vi "Pointer producer consumer Read Write Serial Port.vi"(7 "write string":string, 8 "error in (no error)":errorcluster, 11 "VISA resource name out":refnum<visa-resource-name>) -> (0 "error out":errorcluster, 1 "timeout?":bool, 2 "read string":string, 3 "bytes read":u32)   [LabVIEW 2014]
doc: "The Basic Serial Read and Write example performs a Serial Port Read, a Serial Port Write, or a combination of these actions. The user selects the actions (read or write) on the front panel. If both are selected, the VI will write the data first, read data, and then close the VISA session that is opened to the port. This VI will wait until the specified number of bytes is received at the port or until a termination character is read.\n\nINSTRUCTIONS:\n1) Select the serial resource and configuration parameters (baud rate, data bits, parity, stop bits, flow control).\n2) Select the operations to be performed. \n3) Connect the serial port to your device. If no device is available, perform a loopback test by doing one of the following. Short pins 2 and 3 on a RS-232 cable or short pin 4 to pin 8 and pin 5 to pin 9 on a RS-485/422 cable. \n4) Run the VI to see the data read. (The \"read string\" will match the \"string to write\" if a loopback test was performed.)\n\nNote: The parameters set for the serial port must match the parameters of the connected instrument or device. In this example, the bytes to read parameter specifies the number of bytes that the serial port reads. If there were more bytes at the port than the number specified in bytes to read, those bytes would not be read. Also, if you specify to read more bytes than the number of bytes actually read, you might receive a timeout error message.\n\nOn the block diagram, the Configure Serial Port VI sets the configuration parameters. The front panel displays the controls used to configure the basic parameters, such as baud rate, data bits, and parity. Constants configure the other parameters the user probably does not need set. After the VISA Configure Serial Port VI opens the VISA session and configures the port, the VI passes the VISA resource name to other VIs that perform operations on that VISA resource. The VISA Write function sends a command to the serial device and the VISA Read function returns data based on the command. The VISA Close function then closes the reference to the serial device. It is important to close the reference; otherwise communication through with that port through protocols other than VISA might not be possible."
uses:
  <vilib>/Instr/_visa.llb/VISA Flush IO Buffer Mask.ctl
panel:
  out "comm time":u32
  # "Select the serial resource and the operations (Read, Write, or both) to be performed.  If both are selected, the VI will write the data first, read data and then close the VISA session that is opened to the port.  This VI will wait until the specified number of bytes is received at the port or until a termination character is read."
  # "For additional information select File >> VI Properties >> Documentation"
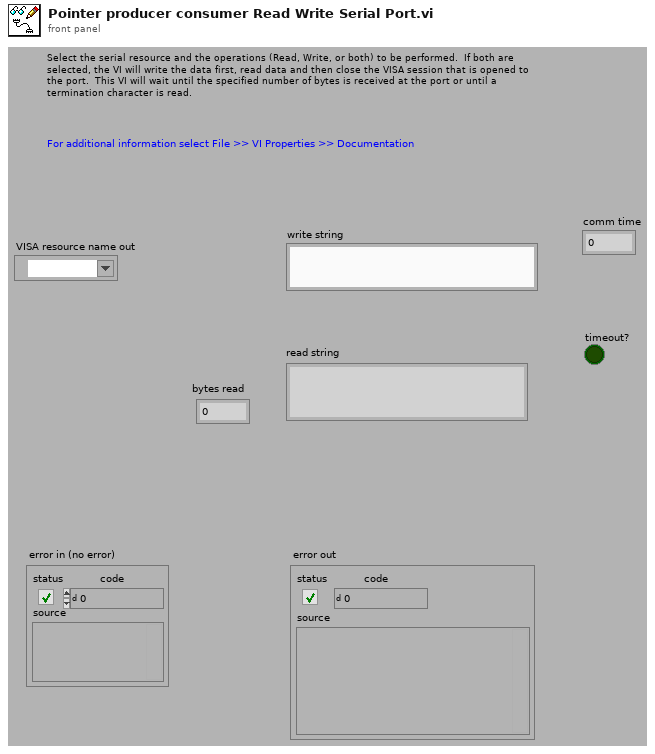
[diagram p1: front panel]
types:
  T1 = typedef "VISA Flush IO Buffer Mask.ctl" = u16
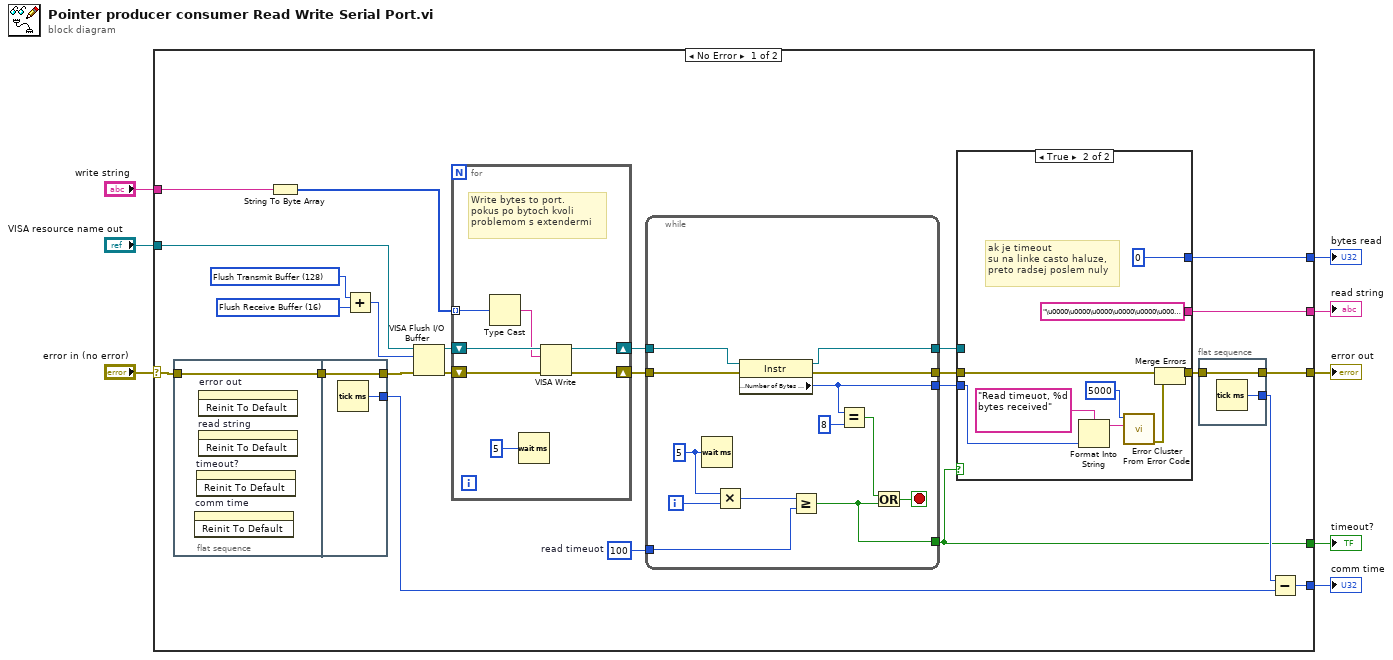
[diagram p0: block diagram]
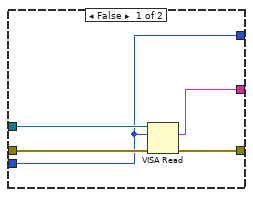
[diagram p2: hidden frame]
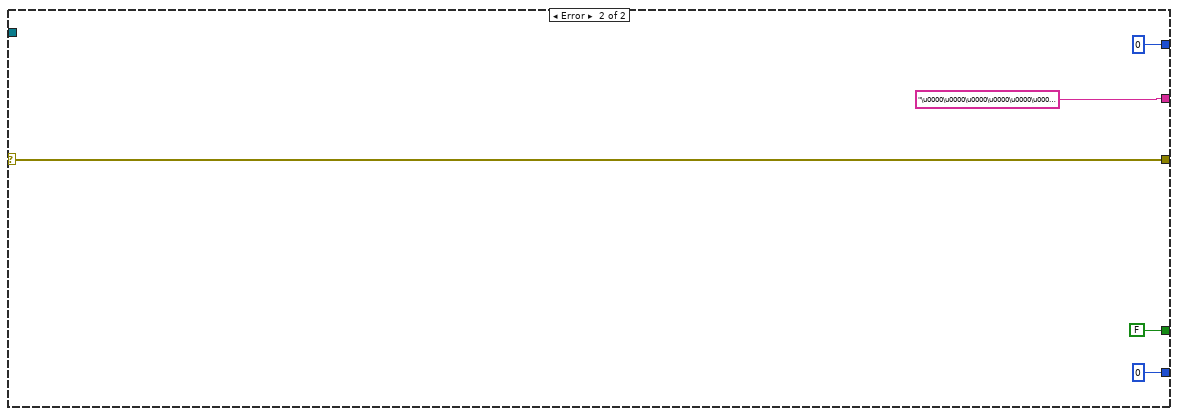
[diagram p3: hidden frame]
diagram:
  n1 = case shown="No Error" "error in (no error)" {
    selector: "error in (no error)" -> [w9 w76]
    tunnel: [w32 u32 0] -> w8
    tunnel: [w29 w76] -> w7
    tunnel: "VISA resource name out" -> [w25 _]
    tunnel: "write string" -> [w15 _]
    tunnel: [w13 FALSE] -> w4
    tunnel: [w12 "\u0000\u0000\u0000\u0000\u0000\u0000\u0000\u0000" ("read buffer")] -> w3
    tunnel: [w11 u32 0 ("Bytes at Port")] -> w2
    frame No Error {
      w16 = u32 100  # read timeuot
      w22 = T1 128 items=["Flush Receive Buffer"=16, "Write Transmit Buffer to Device"=32, "Flush Receive Buffer (No I/O)"=64, "Flush Transmit Buffer"=128] ("Mask")
      w24 = T1 16 items=["Flush Receive Buffer"=16, "Write Transmit Buffer to Device"=32, "Flush Receive Buffer (No I/O)"=64, "Flush Transmit Buffer"=128] ("Mask")
      n2 = flat-sequence {
        tunnel: w9 -> [w56]
        tunnel: [w56] -> w10
        tunnel: [w58] -> w28
        tunnel: [w57] -> w31
        tunnel: w10 -> [w58]
        frame #0 {
          n3 = invoke on="comm time" class="DigNum (strict)" method="Reinit To Default"() -> ()  [unwired: 3 in, 3 out]
          n4 = invoke on="timeout?" class="Bool (strict)" method="Reinit To Default"() -> ()  [unwired: 3 in, 3 out]
          n5 = invoke on="error out" class="Clust (strict)" method="Reinit To Default"() -> ()  [unwired: 3 in, 3 out]
          n6 = invoke on="read string" class="Str" method="Reinit To Default"() -> ()  [unwired: 3 in, 3 out]
        }
        frame #1 {
          n7 = Tick Count (ms)() -> (millisecond timer value=w57:u32)
        }
      }
      n8 = String To Byte Array(string=w15) -> (unsigned byte array=w14:u8[])
      n9 = Add(x=w22, y=w24) -> (x+y=w23:T1)
      n10 = VISA Flush I/O Buffer(VISA resource name=w25, mask (16)=w23, error in (no error)=w28) -> (VISA resource name out=w26:refnum<visa-resource-name>, error out=w27:errorcluster)
      n11 = for {
        shift-right: [w38] -> w21
        shift-left: w27 -> [w40]
        shift-right: [w37] -> w20
        shift-left: w26 -> [w39]
        tunnel: w14 -> [w35] mode=indexing
        # "Write bytes to port.\npokus po bytoch kvoli\nproblemom s extendermi"
        n12 = Type Cast(x=w35) -> (*(type *) &x=w34:string)  [unwired: 1 in]
        n13 = Wait (ms)(milliseconds to wait=u32 5 ("delay before read (ms)")) -> ()  [unwired: 1 out]
        n14 = VISA Write(VISA resource name=w39, write buffer=w34, error in (no error)=w40) -> (VISA resource name out=w37:refnum<visa-resource-name>, error out=w38:errorcluster)  [unwired: 1 out]
      }
      n15 = while {
        tunnel: w21 -> [w53]
        tunnel: w20 -> [w52]
        tunnel: [w51] -> w19
        tunnel: [w50] -> w18
        tunnel: [w48] -> w17
        tunnel: w16 -> [w43]
        tunnel: [w41] -> w13
        i -> [w45]
        stop <- w42 stop-if-true
        w46 = u32 5 ("delay before read (ms)")
        n16 = Wait (ms)(milliseconds to wait=w46) -> ()  [unwired: 1 out]
        n17 = Multiply(x=w46, y=w45) -> (x*y=w44:u32)
        n18 = property class="Instr"(reference=w52, error in=w53) -> (reference out=w50:refnum<visa-resource-name>, error out=w51:errorcluster, "Serial Settings:Number of Bytes at Serial Port"=w48:u32)
        n19 = Greater Or Equal?(x=w44, y=w43) -> (x >= y?=w41:bool)
        n20 = Equal?(x=w48, y=u32 8 ("delay before read (ms)")) -> (x = y?=w47:bool)
        n21 = Or(x=w47, y=w41) -> (x .or. y?=w42:bool)
      }
      n22 = case shown="True" w13 {
        tunnel: w18 -> [w61 _]
        tunnel: [w63 "\u0000\u0000\u0000\u0000\u0000\u0000\u0000\u0000" ("read buffer")] -> w12
        tunnel: w19 -> [w60 w72]
        tunnel: [w62 w69] -> w33
        tunnel: [w59 u32 0 ("Bytes at Port")] -> w11
        tunnel: w17 -> [w59 w66]
        frame False {
          n23 = VISA Read(VISA resource name=w61, byte count=w59, error in (no error)=w60) -> (read buffer=w63:string, error out=w62:errorcluster)  [unwired: 2 out]
        }
        frame True {
          # "ak je timeout\nsu na linke casto haluze,\npreto radsej poslem nuly"
          n24 = Format Into String(format string="Read timeuot, %d bytes received" ("error message (\"\")"), w66) -> (resulting string=w65:string)  [unwired: 2 in, 1 out]
          n25 = call <vilib>:"Error Cluster From Error Code.vi"("error message (\"\")"=w65, "error code (0)"=5000) -> ("error out"=w68:errorcluster)  [unwired: 7 in]
          n26 = Merge Errors(w72, w68) -> (w69:errorcluster)
        }
      }
      n27 = flat-sequence {
        tunnel: [w55] -> w29
        tunnel: w33 -> [w55]
        tunnel: [w54] -> w30
        frame #0 {
          n28 = Tick Count (ms)() -> (millisecond timer value=w54:u32)
        }
      }
      n29 = Subtract(x=w30, y=w31) -> (x-y=w32:u32)
    }
    frame Error {
    }
  }
  "error out" <- w7
  "comm time" <- w8
  "timeout?" <- w4
  "read string" <- w3
  "bytes read" <- w2
